vi "加速度_裕度指标.vi"(10 "峰值":dbl, 11 "信号X":dbl[](array[numeric])) -> (3 "裕度指标":dbl)   [LabVIEW 2014]
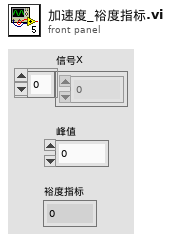
[diagram p1: front panel]
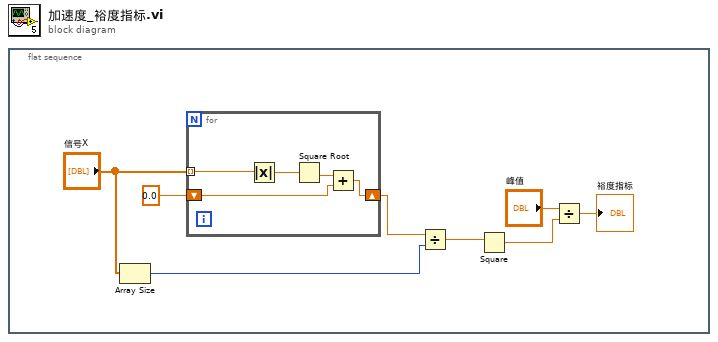
[diagram p0: block diagram]
diagram:
  n1 = flat-sequence {
    frame #0 {
      n2 = Array Size(array="信号X") -> (size(s)=w5:i32)
      n3 = for {
        tunnel: "信号X" -> [w13] mode=indexing
        shift-right: [w9] -> w6
        shift-left: 0.0 -> [w11]
        n4 = Absolute Value(x=w13) -> (abs(x)=w12:dbl)
        n5 = Square Root(x=w12) -> (sqrt(x)=w10:dbl)
        n6 = Add(x=w10, y=w11) -> (x+y=w9:dbl)
      }
      n7 = Divide(x=w6, y=w5) -> (x/y=w4:dbl)
      n8 = Square(x=w4) -> (x^2=w3:dbl)
      n9 = Divide(x="峰值", y=w3) -> (x/y=→"裕度指标":dbl)
    }
  }
